vi "Ejercicio_12_Nodo_de_Propiedad.vi"() -> ()   [LabVIEW 2020]
panel:
  out "Cadena caracteres":string
  out "Boolean":bool
  in  "Posicion Horizontal":dbl(slide) scale=0.0..300.0
  in  "Posicion Vertical":dbl(slide) scale=0.0..300.0
  in  "Deshabilitar":bool
  in  "Límite":dbl
  in  "stop":bool
  out "Tank":dbl(slide) scale=0.0..10.0
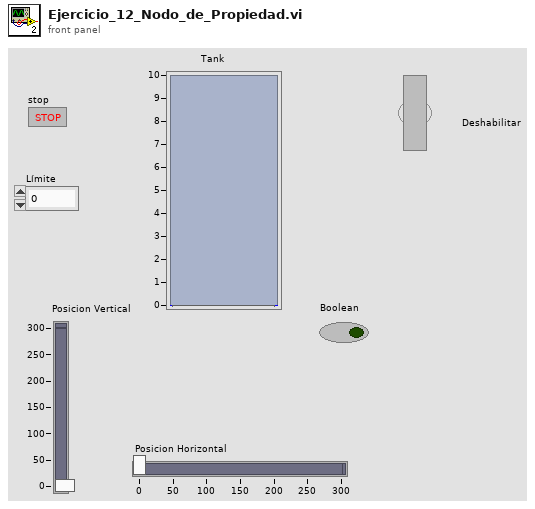
[diagram p1: front panel]
types:
  T1 = cluster{"Posicion Horizontal":dbl, "Posicion Vertical":dbl}
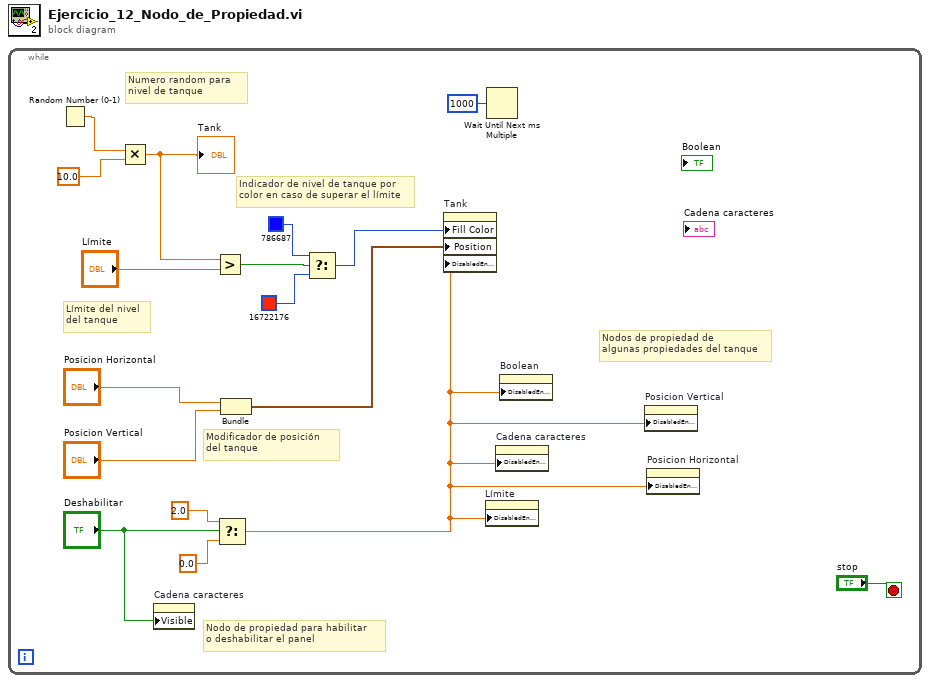
[diagram p0: block diagram]
diagram:
  n1 = while {
    stop <- "stop" stop-if-true
    # "Nodo de propiedad para habilitar \no deshabilitar el panel"
    # "Modificador de posición \ndel tanque"
    # "Indicador de nivel de tanque por \ncolor en caso de superar el límite"
    # "Límite del nivel \ndel tanque"
    # "Nodos de propiedad de \nalgunas propiedades del tanque"
    # "Numero random para \nnivel de tanque"
    n2 = Random Number (0-1)() -> (number: 0 to 1=w16:dbl)
    n3 = Multiply(x=w16, y=10.0) -> (x*y=w13:dbl)
    "Tank" <- w13
    n4 = property on="Cadena caracteres" class="Str"("Visible"="Deshabilitar") -> ()  [unwired: 2 in, 2 out]
    n5 = Greater?(x=w13, y="Límite") -> (0:w12:bool)
    n6 = Select(t=2.0, s="Deshabilitar", f=0.0) -> (s? t:f=w4:dbl)
    n7 = Bundle("Posicion Horizontal"="Posicion Horizontal", "Posicion Vertical"="Posicion Vertical") -> (w7:T1)  [unwired: 1 in]
    n8 = Select(t=u32 786687, s=w12, f=u32 16722176) -> (s? t:f=w8:u32)
    n9 = property on="Tank" class="Slide (strict)"("Fill Color"=w8, "Position"=w7, "DisabledEnum"=w4) -> ()  [unwired: 2 in, 2 out]
    n10 = property on="Límite" class="DigNum (strict)"("DisabledEnum"=w4) -> ()  [unwired: 2 in, 2 out]
    n11 = Wait Until Next ms Multiple(millisecond multiple=u32 1000) -> ()  [unwired: 1 out]
    n12 = property on="Cadena caracteres" class="Str"("DisabledEnum"=w4) -> ()  [unwired: 2 in, 2 out]
    n13 = property on="Boolean" class="Bool (strict)"("DisabledEnum"=w4) -> ()  [unwired: 2 in, 2 out]
    n14 = property on="Posicion Vertical" class="Slide (strict)"("DisabledEnum"=w4) -> ()  [unwired: 2 in, 2 out]
    n15 = property on="Posicion Horizontal" class="Slide (strict)"("DisabledEnum"=w4) -> ()  [unwired: 2 in, 2 out]
  }
